vi "main.vi"() -> ()   [LabVIEW 2012]
uses:
  Typedefs/Control 1.ctl
  Typedefs/Control 2.ctl
  OpenConnection/OpenConnectionInstances/OpenConnection_Control1.vi
  ReadValue/ReadValueInstances/ReadValue_Control1.vi
  OpenConnection/OpenConnectionInstances/OpenConnection_Control2.vi
  ReadValue/ReadValueInstances/ReadValue_Control2.vi
  WriteValue/WriteValueInstances/WriteValue_Control1.vi
  WriteValue/WriteValueInstances/WriteValue_Control2.vi
panel:
  out "value 2":T1
  out "value":T2
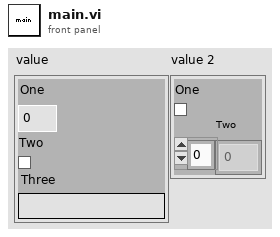
[diagram p1: front panel]
types:
  T1 = typedef "Control 2.ctl" = cluster{"One":bool, "Two":i32[]}
  T2 = typedef "Control 1.ctl" = cluster{"One":dbl, "Two":bool, "Three":string}
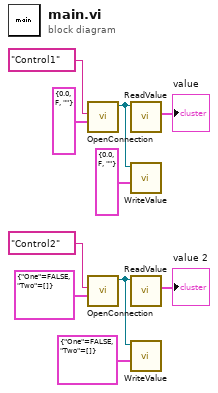
[diagram p0: block diagram]
diagram:
  n1 = call-poly "OpenConnection.vi"("type"=T2 {"One"=0.0, "Two"=FALSE, "Three"=""} ("Cluster1"), "topicName"="Control1") -> ("reference"=w1:refnum<vi>)  [unwired: 8 in, 1 out]
  n2 = call-poly "OpenConnection.vi"("type"=T1 {"One"=FALSE, "Two"=[]} ("Control 2"), "topicName"="Control2") -> ("reference"=w2:refnum<vi>)  [unwired: 8 in, 1 out]
  n3 = call-poly "ReadValue.vi"("reference"=w1) -> ("value"=→"value":T2)  [unwired: 10 in]
  n4 = call-poly "WriteValue.vi"("value"=T2 {"One"=0.0, "Two"=FALSE, "Three"=""}, "reference"=w1) -> ()  [unwired: 10 in]
  n5 = call-poly "ReadValue.vi"("reference"=w2) -> ("value"=→"value 2":T1)  [unwired: 10 in]
  n6 = call-poly "WriteValue.vi"("value"=T1 {"One"=FALSE, "Two"=[]}, "reference"=w2) -> ()  [unwired: 10 in]
